vi "Delayed Tree Update.vi"(8 "error in (no error)":errorcluster, 11 "Actor Monitor in":refnum<class "Actor Monitor.lvclass">) -> (0 "error out":errorcluster, 3 "Actor Monitor out":refnum<class "Actor Monitor.lvclass">)   [LabVIEW 2018, in "Monitored Actor.lvlib" / "Actor Monitor.lvclass"]
doc: "This will queue up a low priority messages to redraw the tree if needed\n\nCopyright: MGI\nAuthored by: Derek Trepanier"
uses:
  Actor Monitor.lvclass
  C:/Program Files (x86)/National Instruments/LabVIEW 2018/vi.lib/ActorFramework/Actor/Actor.lvclass
  Actor Monitor.lvclass/Actor Monitor.ctl
  <vilib>/ActorFramework/Message Enqueuer/Message Priority.ctl
  <vilib>/ActorFramework/Actor/Actor.lvclass/Actor.ctl
  <vilib>/ActorFramework/Message Enqueuer/Message Enqueuer.lvclass/Message Enqueuer.ctl
  <vilib>/ActorFramework/Message Enqueuer/Init from Existing Queue.vi
  <vilib>/ActorFramework/Message Enqueuer/Enqueue.vi
  Actor Monitor Messages/Redraw Tree Msg/Redraw Tree Msg.lvclass
  C:/Program Files (x86)/National Instruments/LabVIEW 2018/vi.lib/ActorFramework/Message/Message.lvclass
  <vilib>/ActorFramework/Message Priority Queue/Priority Enqueue.vi
  <vilib>/ActorFramework/Message Enqueuer/Message Enqueuer.lvclass
  <vilib>/ActorFramework/Actor/Actor.lvclass
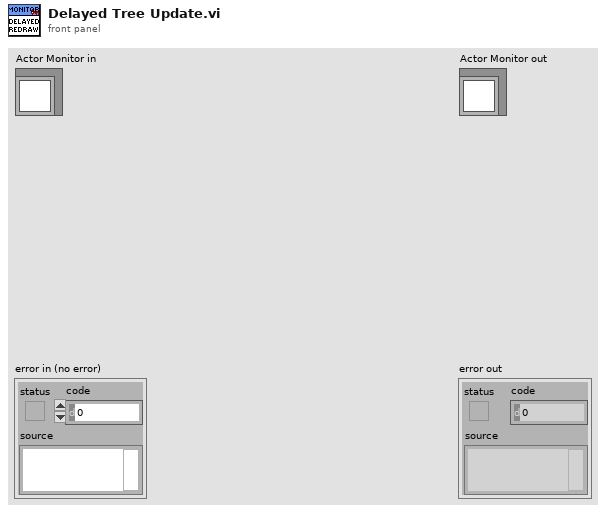
[diagram p1: front panel]
types:
  T1 = typedef "Actor Framework.lvlib/Message Enqueuer.lvclass/Message Priority.ctl" = enum16{"Low", "Normal", "High"}
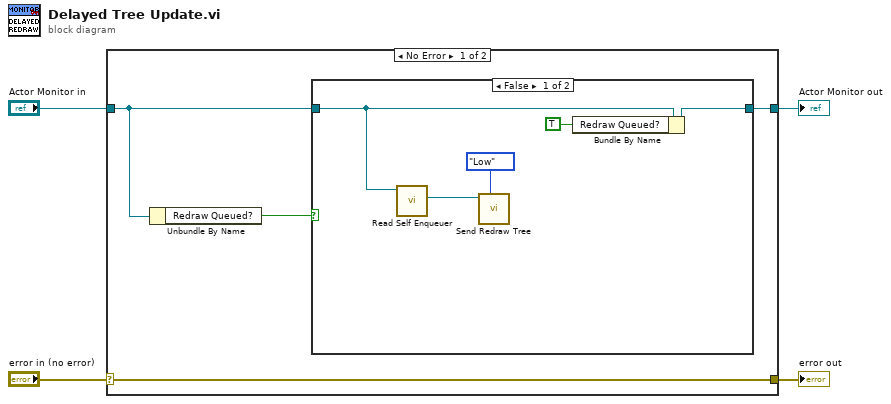
[diagram p0: block diagram]
diagram:
  n1 = case shown="No Error" "error in (no error)" {
    selector: "error in (no error)" -> [w5 w16]
    tunnel: [w5 w16] -> w3
    tunnel: [w8 w15] -> w1
    tunnel: "Actor Monitor in" -> [w7 w15]
    frame No Error {
      n2 = Unbundle By Name(w7) -> ("Redraw Queued?"=w6:bool)
      n3 = case shown="False" w6 {
        tunnel: [w10 w14] -> w8
        tunnel: w7 -> [w12 w14]
        frame False {
          n4 = call <vilib>:"Read Self Enqueuer.vi"("Actor"=w12) -> ("Self Enqueuer"=w11:refnum<class "Message Enqueuer.lvclass">)  [unwired: 10 in]
          n5 = call "Send Redraw Tree.vi"("Message Priority (Normal)"=Message_Priority."Low", "Message Enqueuer"=w11) -> ()  [unwired: 8 in, 2 out]
          n6 = Bundle By Name(cluster=w12, "Redraw Queued?"=TRUE ("Redraw When Idle")) -> (w10:refnum<class "Actor Monitor.lvclass">)
        }
        frame True {
          # "Redraw already queued, don't need to do anything"
        }
      }
    }
    frame Error {
    }
  }
  "error out" <- w3
  "Actor Monitor out" <- w1
